vi "Send Data SubVI.vi"(0 "Data Pin Task In":refnum<k21>, 1 "Sync Pin Task In":refnum<k21>, 2 "Write Pin Task In":refnum<k21>, 3 "Clear Pin Task In":refnum<k21>, 5 "Data":bool[](array[boolean])) -> (6 "Data Pin Task Out":refnum<k21>, 7 "Sync Pin Task Out":refnum<k21>, 8 "Write Pin Task Out":refnum<k21>, 9 "Clear Pin Task Out":refnum<k21>)   [LabVIEW 2020]
uses:
  <vilib>/DAQmx/write.llb/DAQmx Write (Digital Bool 1Line 1Point).vi
  <vilib>/DAQmx/miscellaneous.llb/DAQmx Fill In Error Info.vi
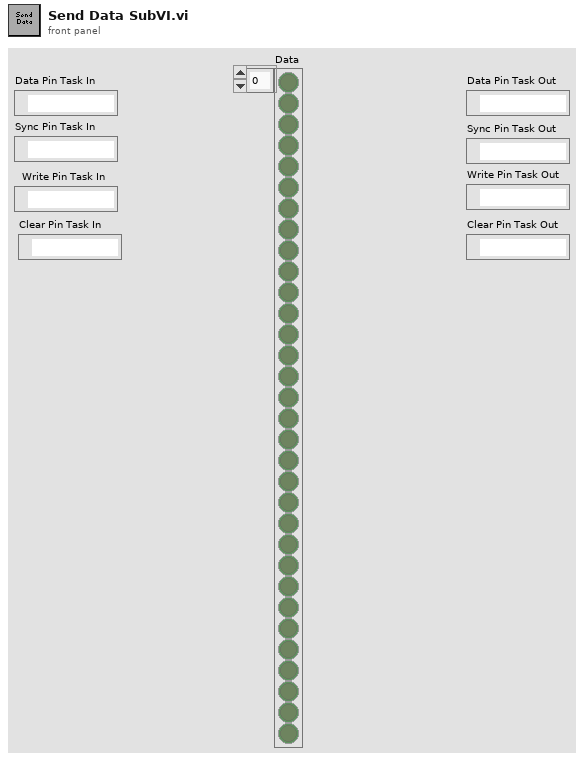
[diagram p1: front panel]
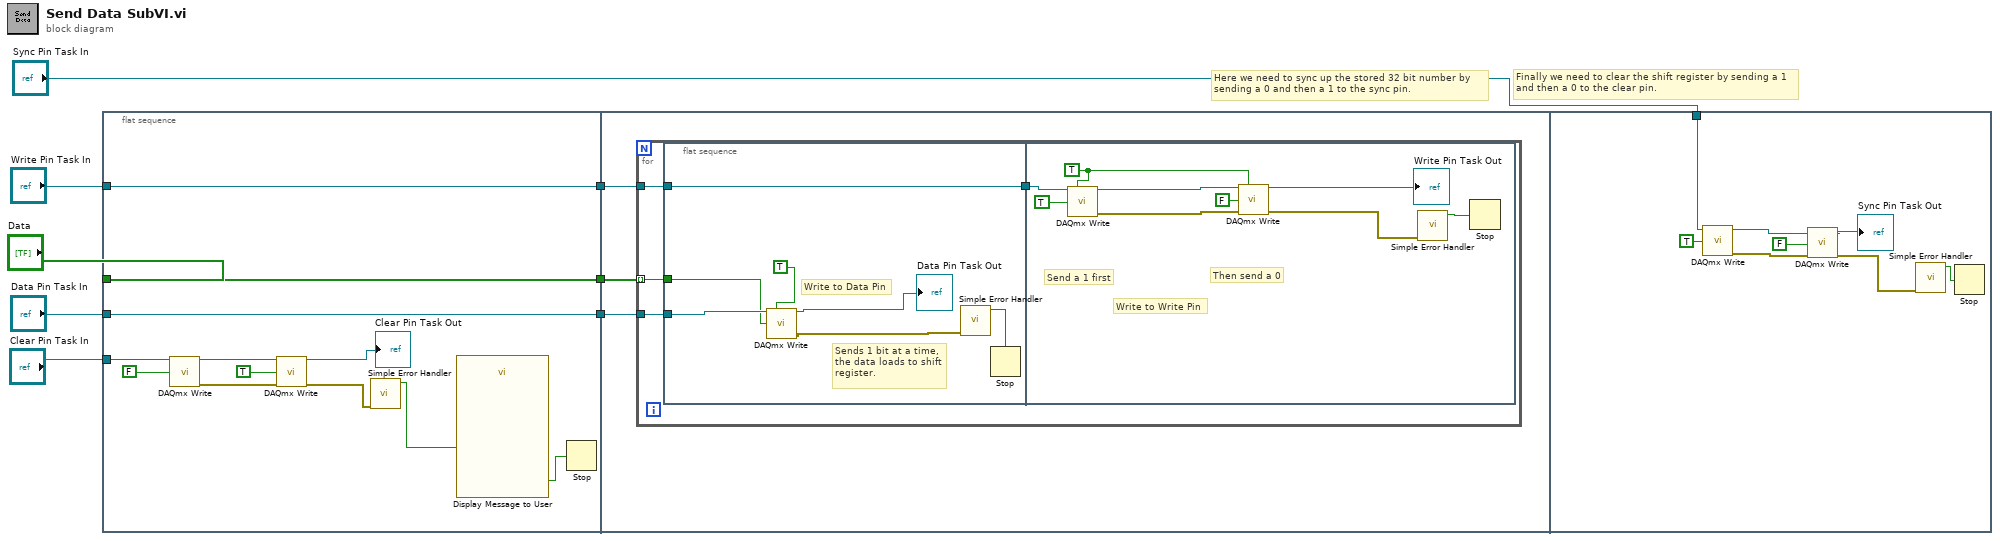
[diagram p0: block diagram]
diagram:
  # "Finally we need to clear the shift register by sending a 1\nand then a 0 to the clear pin."
  # "Here we need to sync up the stored 32 bit number by \nsending a 0 and then a 1 to the sync pin."
  n1 = flat-sequence {
    tunnel: "Data" -> [w18]
    tunnel: "Data Pin Task In" -> [w19]
    tunnel: "Write Pin Task In" -> [w20]
    tunnel: [w20] -> w6
    tunnel: [w19] -> w5
    tunnel: [w18] -> w4
    tunnel: "Clear Pin Task In" -> [w11]
    tunnel: w6 -> [w23]
    tunnel: w5 -> [w22]
    tunnel: w4 -> [w21]
    tunnel: "Sync Pin Task In" -> [w45]
    frame #0 {
      n2 = call-poly <vilib>:"DAQmx Write.vi"("task/channels in"=w11, "data"=FALSE) -> ("task out"=w15:refnum<k21>, "error out"=w14:errorcluster)  [unwired: 11 in, 1 out]
      n3 = call-poly <vilib>:"DAQmx Write.vi"("task/channels in"=w15, "data"=TRUE, "error in"=w14) -> ("task out"=→"Clear Pin Task Out":refnum<k21>, "error out"=w12:errorcluster)  [unwired: 10 in, 1 out]
      n4 = call <vilib>:"Simple Error Handler.vi"("error in (no error)"=w12) -> ("error?"=w10:bool)  [unwired: 4 in, 4 out]
      n5 = call "Display Message to User"("Enable"=w10) -> ("OK"=w9:bool)  [unwired: 9 in, 1 out]
      n6 = Stop(stop? (T)=w9) -> ()
    }
    frame #1 {
      n7 = for {
        tunnel: w23 -> [w27]
        tunnel: w22 -> [w25]
        tunnel: w21 -> [w24] mode=indexing
        n8 = flat-sequence {
          tunnel: w27 -> [w34]
          tunnel: [w34] -> w26
          tunnel: w25 -> [w33]
          tunnel: w24 -> [w32]
          tunnel: w26 -> [w41]
          frame #0 {
            # "Sends 1 bit at a time,\nthe data loads to shift\nregister."
            # "Write to Data Pin"
            n9 = call-poly <vilib>:"DAQmx Write.vi"("task/channels in"=w33, "auto start"=TRUE, "data"=w32) -> ("task out"=→"Data Pin Task Out":refnum<k21>, "error out"=w29:errorcluster)  [unwired: 10 in, 1 out]
            n10 = call <vilib>:"Simple Error Handler.vi"("error in (no error)"=w29) -> ("error?"=w28:bool)  [unwired: 4 in, 4 out]
            n11 = Stop(stop? (T)=w28) -> ()
          }
          frame #1 {
            w36 = TRUE
            # "Then send a 0"
            # "Send a 1 first"
            # "Write to Write Pin"
            n12 = call-poly <vilib>:"DAQmx Write.vi"("task/channels in"=w41, "auto start"=w36, "data"=TRUE) -> ("task out"=w37:refnum<k21>, "error out"=w38:errorcluster)  [unwired: 10 in, 1 out]
            n13 = call-poly <vilib>:"DAQmx Write.vi"("task/channels in"=w37, "auto start"=w36, "data"=FALSE, "error in"=w38) -> ("task out"=→"Write Pin Task Out":refnum<k21>, "error out"=w39:errorcluster)  [unwired: 9 in, 1 out]
            n14 = call <vilib>:"Simple Error Handler.vi"("error in (no error)"=w39) -> ("error?"=w35:bool)  [unwired: 4 in, 4 out]
            n15 = Stop(stop? (T)=w35) -> ()
          }
        }
      }
    }
    frame #2 {
      n16 = call-poly <vilib>:"DAQmx Write.vi"("task/channels in"=w45, "data"=TRUE) -> ("task out"=w46:refnum<k21>, "error out"=w47:errorcluster)  [unwired: 11 in, 1 out]
      n17 = call-poly <vilib>:"DAQmx Write.vi"("task/channels in"=w46, "data"=FALSE, "error in"=w47) -> ("task out"=→"Sync Pin Task Out":refnum<k21>, "error out"=w48:errorcluster)  [unwired: 10 in, 1 out]
      n18 = call <vilib>:"Simple Error Handler.vi"("error in (no error)"=w48) -> ("error?"=w44:bool)  [unwired: 4 in, 4 out]
      n19 = Stop(stop? (T)=w44) -> ()
    }
  }
